vi "Configure Hardware.vi"(8 "error in (no error)":errorcluster, 11 "Hardware Resources in":T1) -> (0 "error out":errorcluster, 3 "Hardware Resources out":T1)   [LabVIEW 2017, in "Acquisition.lvlib"]
doc: "Configure the hardware."
uses:
  Acquisition.lvlib
  Hardware Configuration.ctl
  <vilib>/DAQmx/create/channels.llb/DAQmx Create Channel (AI-Voltage-Basic).vi
  <vilib>/DAQmx/configure/timing.llb/DAQmx Timing (Sample Clock).vi
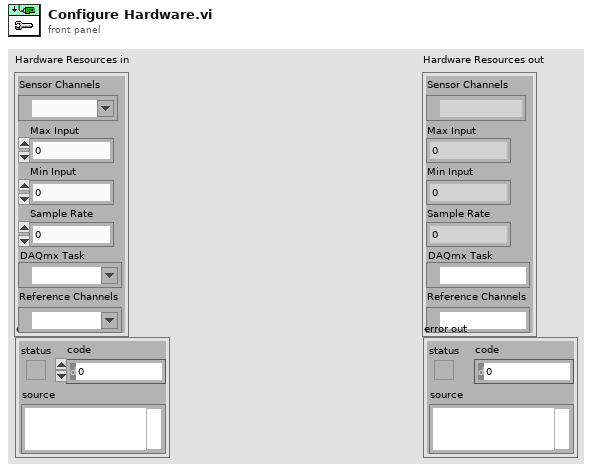
[diagram p1: front panel]
types:
  T1 = typedef "Acquisition.lvlib/Hardware Configuration.ctl" = cluster{"Sensor Channels":tag, "Max Input":dbl, "Min Input":dbl, "Sample Rate":dbl, "DAQmx Task":refnum<k21>, "Reference Channels":tag}
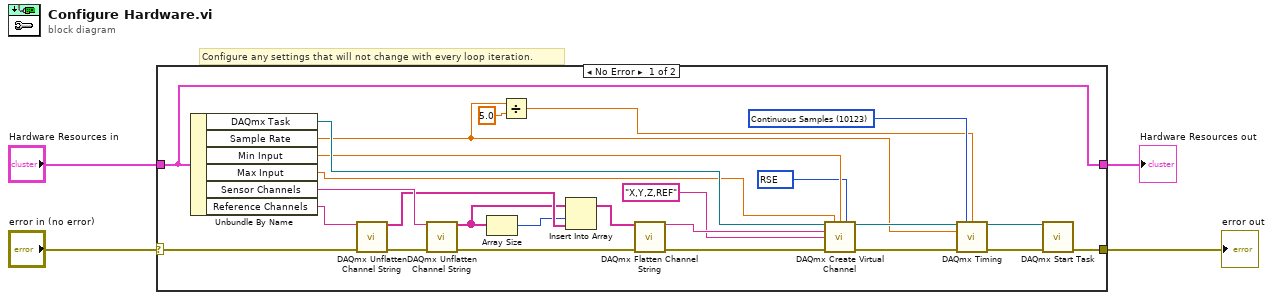
[diagram p0: block diagram]
diagram:
  # "Configure any settings that will not change with every loop iteration."
  n1 = case shown="No Error" "error in (no error)" {
    selector: "error in (no error)" -> [w15 w31]
    tunnel: [w18 w31] -> w3
    tunnel: "Hardware Resources in" -> [w25 w32]
    tunnel: [w25 w32] -> w1
    frame No Error {
      w17 = 10083 items=["Default"=-1, "RSE"=10083, "NRSE"=10078, "Differential"=10106, "Pseudodifferential"=12529] ("input terminal configuration")
      w24 = 10123 items=["Finite Samples"=10178, "Continuous Samples"=10123, "Hardware Timed Single Point"=12522] ("sample mode")
      n2 = Unbundle By Name(w25) -> ("DAQmx Task"=w30:refnum<k21>, "Sample Rate"=w23:dbl, "Min Input"=w28:dbl, "Max Input"=w29:dbl, "Sensor Channels"=w16:tag, "Reference Channels"=w5:tag)
      n3 = call <vilib>:"DAQmx Unflatten Channel String.vi"("names in"=w5, "error in"=w15) -> ("names out"=w13:string[], "error out"=w14:errorcluster)  [unwired: 12 in]
      n4 = call <vilib>:"DAQmx Unflatten Channel String.vi"("names in"=w16, "error in"=w14) -> ("names out"=w11:string[], "error out"=w9:errorcluster)  [unwired: 12 in]
      n5 = Array Size(array=w11) -> (size(s)=w12:i32)
      n6 = Divide(x=w23, y=5.0) -> (x/y=w21:dbl)
      n7 = Insert Into Array(array=w11, index=w12, new element=w13) -> (w10:string[])
      n8 = call <vilib>:"DAQmx Flatten Channel String.vi"("names in"=w10, "error in"=w9) -> ("names out"=w7:string, "error out"=w8:errorcluster)  [unwired: 12 in]
      n9 = call-poly <vilib>:"DAQmx Create Virtual Channel.vi"("task in"=w30, "maximum value"=w29, "minimum value"=w28, "input terminal configuration"=w17, "physical channels"=w7, "name to assign"="X,Y,Z,REF", "error in"=w8) -> ("task out"=w27:refnum<k21>, "error out"=w26:errorcluster)  [unwired: 7 in]
      n10 = call-poly <vilib>:"DAQmx Timing.vi"("task/channels in"=w27, "sample mode"=w24, "samples per channel"=w21, "rate"=w23, "error in"=w26) -> ("task out"=w19:refnum<k21>, "error out"=w20:errorcluster)  [unwired: 9 in]
      n11 = call <vilib>:"DAQmx Start Task.vi"("task/channels in"=w19, "error in"=w20) -> ("error out"=w18:errorcluster)  [unwired: 12 in, 1 out]
    }
    frame Error {
    }
  }
  "Hardware Resources out" <- w1
  "error out" <- w3
